vi "StateMachine.vi"() -> ()   [LabVIEW 2021]
uses:
  SynchroCheckCentral.ctl
  SynchroCheckCentral_Info.ctl
  SynchroCheckCentral_Data.ctl
  AFE_froming_Central.ctl
  AFE_froming_Central_Info.ctl
  AFE_froming_Central_Data.ctl
  General Purpose/references.ctl
  Connected_OPF.ctl
  Connected_OPF_Info.ctl
  Connected_OPF_Data.ctl
  Optimal_slack_selection.ctl
  Optimal_slack_selection_Info.ctl
  Optimal_slack_selection_Data.ctl
  State Machine.ctl
panel:
  in  "IN AFE":T1={"Info"={"Resource"="Zenone", "Problem"=FALSE, "Timestamp"=0.0}, "Data"={"Start forming 1"=FALSE, "Forming/Following"=[], "Start forming 2"=FALSE, "measurements"={"Vdc1"=0.0, "P1"=0.0, "Vdc2"=0.0, "P2"=0.0, "Q2"=0.0, "Vdc3"=0.0, "P3"=0.0, "Q3"=0.0, "Vdc4"=0.0, "P4"=0.0, "Q4"=0.0, "Q1"=0.0}, "Status"=[], "references"={"Vdc1"=0.0, "Vdc2"=0.0, "Qac2"=0.0, "Vdc3"=0.0, "Qac3"=0.0, "Vdc4"=0.0, "Qac4"=0.0, "Qac1"=0.0, "V_arg2"=0.0, "V_abs2"=0.0, "V_abs1"=0.0, "V_arg1"=0.0, "freq1"=0.0, "freq2"=0.0}}}
  in  "IN cOPF":T5={"Info"={"Resource"="Zenone", "Problem"=FALSE, "Timestamp"=0.0}, "Data"={"Operation mode"="Grid connected", "solution feasible"=FALSE, "Optimal slack"="AFE 1", "setpoints"=[]}}
  in  "IN iOPF":T5={"Info"={"Resource"="Zenone", "Problem"=FALSE, "Timestamp"=0.0}, "Data"={"Operation mode"="Grid connected", "solution feasible"=FALSE, "Optimal slack"="AFE 1", "setpoints"=[]}}
  in  "IN slack":T8={"Info"={"Resource"="Zenone", "Problem"=FALSE, "Timestamp"=0.0}, "Data"={"Operation mode"="Grid connected", "Optimal slack"="AFE 1", "Time-To-Live"=0.0}}
  in  "IN synchro":T11={"Info"={"Resource"="SyncroCheck", "Problem"=FALSE, "Timestamp"=0.0}, "Data"={"close/open relay"=TRUE, "Operation mode"="Grid connected", "Frequency"=0.0, "Angle"=0.0, "Magnitude"=0.0, "synchronised"=TRUE}}
  out "OUT iOPF":T5={"Info"={"Resource"="Zenone", "Problem"=FALSE, "Timestamp"=0.0}, "Data"={"Operation mode"="Grid connected", "solution feasible"=FALSE, "Optimal slack"="AFE 1", "setpoints"=[]}}
  out "OUT cOPF":T5={"Info"={"Resource"="Zenone", "Problem"=FALSE, "Timestamp"=0.0}, "Data"={"Operation mode"="Grid connected", "solution feasible"=FALSE, "Optimal slack"="AFE 1", "setpoints"=[]}}
  out "OUT AFE":T1={"Info"={"Resource"="Zenone", "Problem"=FALSE, "Timestamp"=0.0}, "Data"={"Start forming 1"=FALSE, "Forming/Following"=[], "Start forming 2"=FALSE, "measurements"={"Vdc1"=0.0, "P1"=0.0, "Vdc2"=0.0, "P2"=0.0, "Q2"=0.0, "Vdc3"=0.0, "P3"=0.0, "Q3"=0.0, "Vdc4"=0.0, "P4"=0.0, "Q4"=0.0, "Q1"=0.0}, "Status"=[], "references"={"Vdc1"=0.0, "Vdc2"=0.0, "Qac2"=0.0, "Vdc3"=0.0, "Qac3"=0.0, "Vdc4"=0.0, "Qac4"=0.0, "Qac1"=0.0, "V_arg2"=0.0, "V_abs2"=0.0, "V_abs1"=0.0, "V_arg1"=0.0, "freq1"=0.0, "freq2"=0.0}}}
  out "OUT Synchro":T11={"Info"={"Resource"="SyncroCheck", "Problem"=FALSE, "Timestamp"=0.0}, "Data"={"close/open relay"=TRUE, "Operation mode"="Grid connected", "Frequency"=0.0, "Angle"=0.0, "Magnitude"=0.0, "synchronised"=TRUE}}
  out "Time-To-Live (minutes)":dbl
  out "setpoints":dbl[](array[numeric])
  in  "nb instances":i16=7
  out "optimal_slack":string(combo)="AFE 1"
  out "iOPF valid":bool
  out "forming?":bool
  out "cOPF valid?":bool
  out "synchronised?":bool
  in  "to grid connection":bool
  in  "to prepare for grid connection":bool
  in  "to island":bool
  in  "Stop":bool
  in  "to prepare for island":bool
  # "Islanding Manoeuvre - State Machine"
  # "synchronised"
  # "opf connected OK"
  # "opf island OK"
  # "forming?"
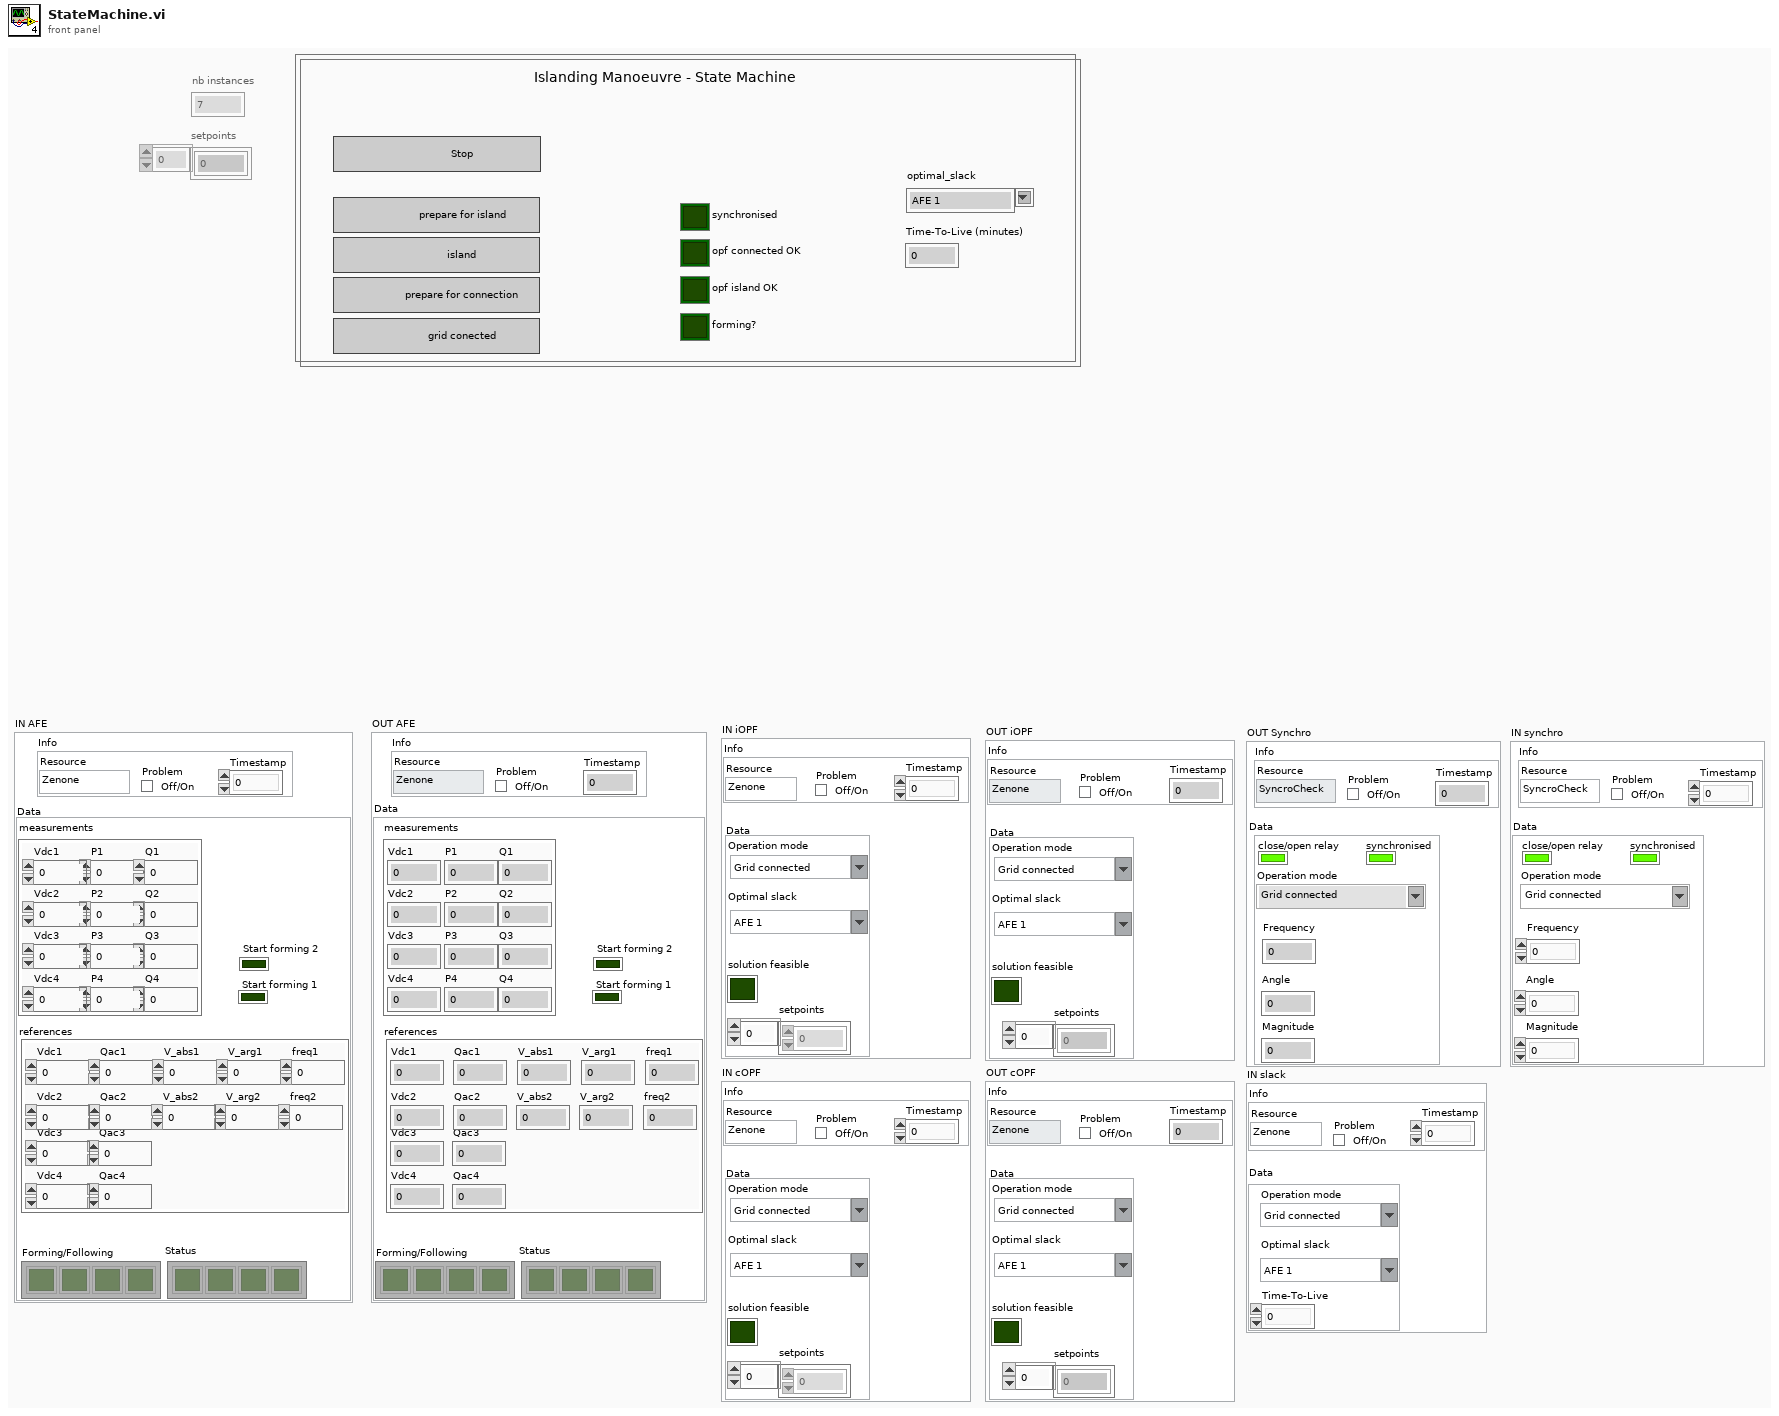
[diagram p1: front panel]
types:
  T1 = typedef "AFE_froming_Central.ctl" = cluster{"Info":T2, "Data":T3}
  T2 = typedef "AFE_froming_Central_Info.ctl" = cluster{"Resource":string, "Problem":bool, "Timestamp":dbl}
  T3 = typedef "AFE_froming_Central_Data.ctl" = cluster{"Start forming 1":bool, "Forming/Following":bool[], "Start forming 2":bool, "measurements":cluster{"Vdc1":dbl, "P1":dbl, "Vdc2":dbl, "P2":dbl, "Q2":dbl, "Vdc3":dbl, "P3":dbl, "Q3":dbl, "Vdc4":dbl, "P4":dbl, "Q4":dbl, "Q1":dbl}, "Status":bool[], "references":T4}
  T4 = typedef "references.ctl" = cluster{"Vdc1":dbl, "Vdc2":dbl, "Qac2":dbl, "Vdc3":dbl, "Qac3":dbl, "Vdc4":dbl, "Qac4":dbl, "Qac1":dbl, "V_arg2":dbl, "V_abs2":dbl, "V_abs1":dbl, "V_arg1":dbl, "freq1":dbl, "freq2":dbl}
  T5 = typedef "Connected_OPF.ctl" = cluster{"Info":T6, "Data":T7}
  T6 = typedef "Connected_OPF_Info.ctl" = cluster{"Resource":string, "Problem":bool, "Timestamp":dbl}
  T7 = typedef "Connected_OPF_Data.ctl" = cluster{"Operation mode":string, "solution feasible":bool, "Optimal slack":string, "setpoints":dbl[]}
  T8 = typedef "Optimal_slack_selection.ctl" = cluster{"Info":T9, "Data":T10}
  T9 = typedef "Optimal_slack_selection_Info.ctl" = cluster{"Resource":string, "Problem":bool, "Timestamp":dbl}
  T10 = typedef "Optimal_slack_selection_Data.ctl" = cluster{"Operation mode":string, "Optimal slack":string, "Time-To-Live":dbl}
  T11 = typedef "SynchroCheckCentral.ctl" = cluster{"Info":T12, "Data":T13}
  T12 = typedef "SynchroCheckCentral_Info.ctl" = cluster{"Resource":string, "Problem":bool, "Timestamp":dbl}
  T13 = typedef "SynchroCheckCentral_Data.ctl" = cluster{"close/open relay":bool, "Operation mode":string, "Frequency":dbl, "Angle":dbl, "Magnitude":dbl, "synchronised":bool}
  T14 = typedef "State Machine.ctl" = enum16{"Grid connected", "Prepare for island", "Island", "Prepare for connection"}
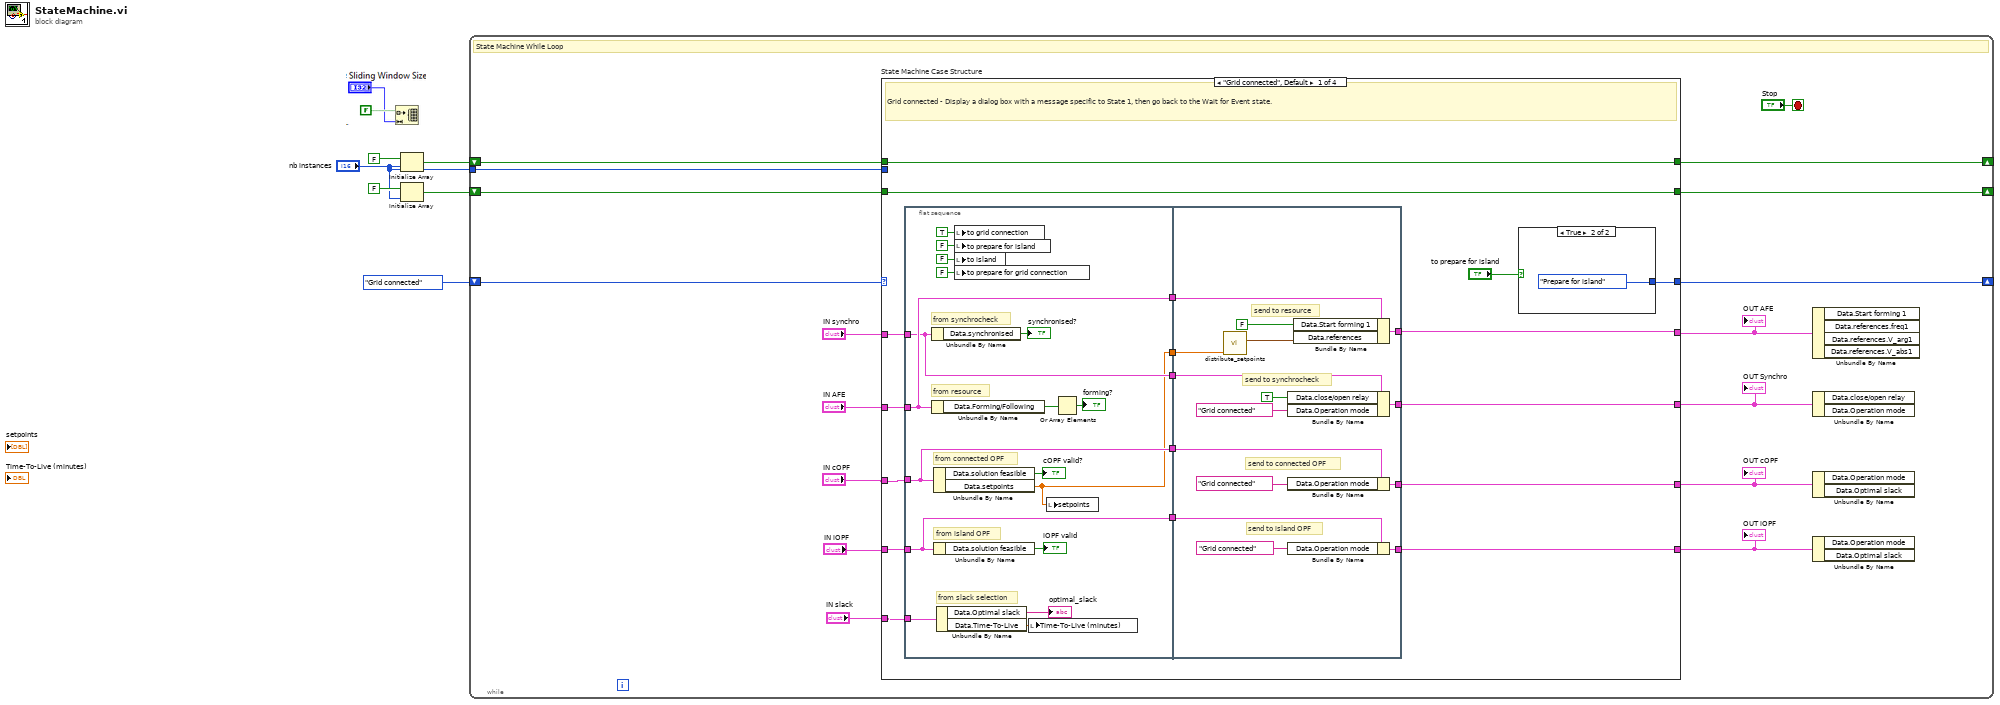
[diagram p0: block diagram]
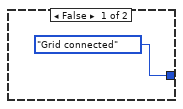
[diagram p2: hidden frame]
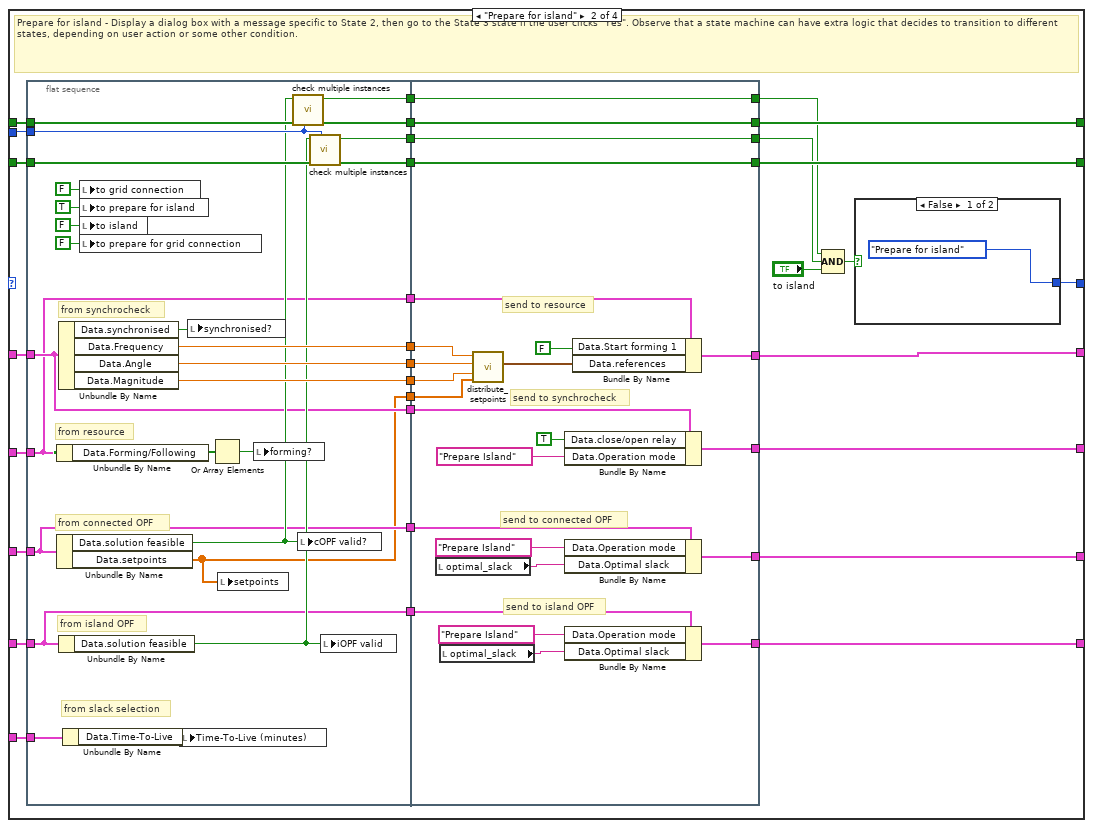
[diagram p3: hidden frame]
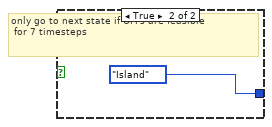
[diagram p4: hidden frame]
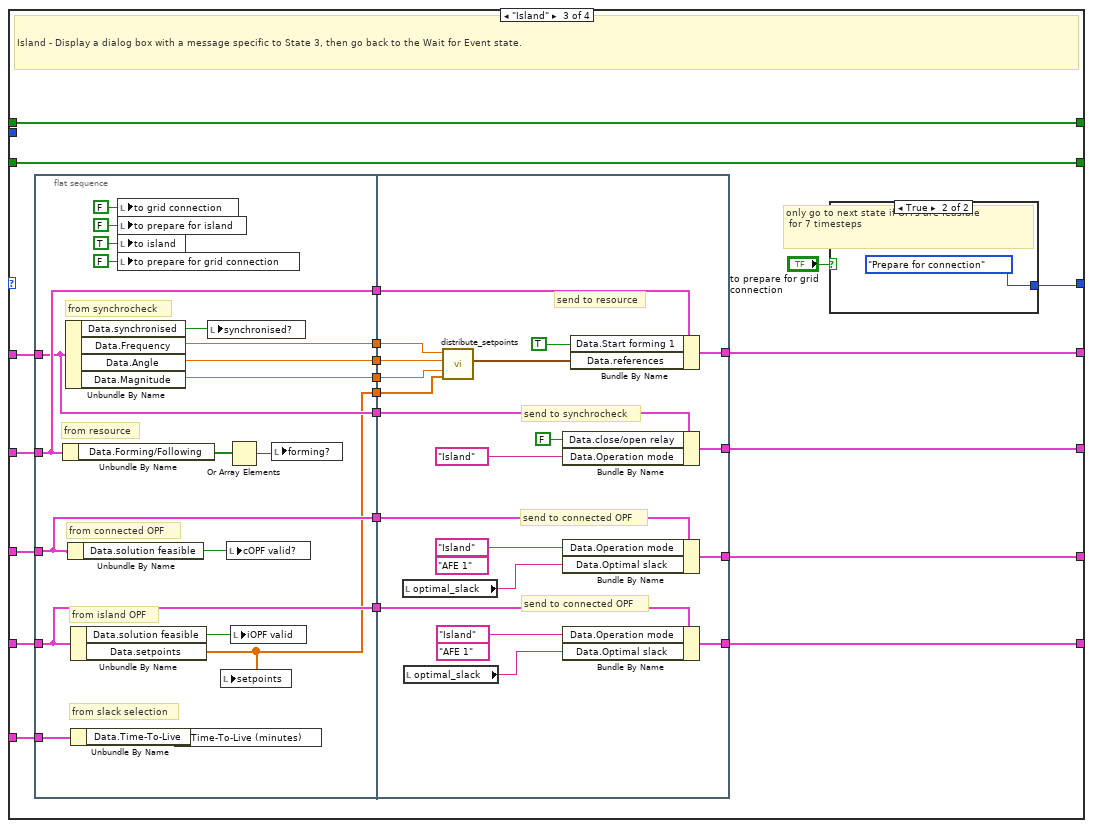
[diagram p5: hidden frame]
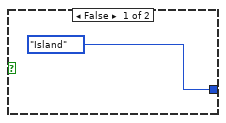
[diagram p6: hidden frame]
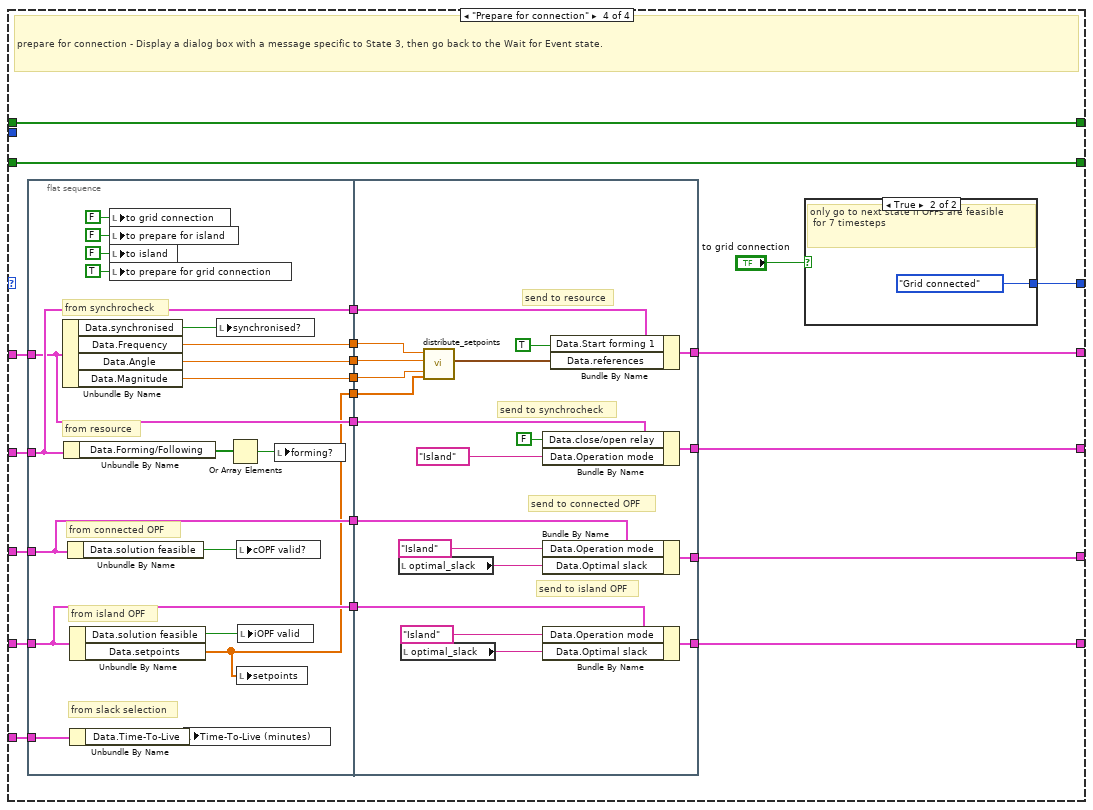
[diagram p7: hidden frame]
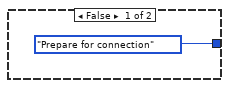
[diagram p8: hidden frame]
diagram:
  n1 = Initialize Array(FALSE, "nb instances") -> (w5:bool[])
  n2 = Initialize Array(FALSE, "nb instances") -> (w3:bool[])
  n3 = while {
    shift-right: [w22] -> _
    shift-left: w5 -> [w23]
    shift-right: [w20] -> _
    shift-left: w3 -> [w21]
    tunnel: "nb instances" -> [w19]
    shift-right: [w12] -> _
    shift-left: State_Machine."Grid connected" ("State") -> [w13]
    stop <- "Stop" stop-if-true
    # "State Machine While Loop"
    n4 = case "State Machine Case Structure" shown="\"Grid connected\", Default" w13 {
      tunnel: "IN synchro" -> [w41 w103 w175 w241]
      tunnel: "IN AFE" -> [w40 w104 w176 w240]
      tunnel: "IN cOPF" -> [w39 w105 w177 w239]
      tunnel: "IN iOPF" -> [w38 w106 w178 w238]
      tunnel: "IN slack" -> [w37 w97 w179 w237]
      tunnel: w23 -> [w36 w102 w174 w236]
      tunnel: [w36 w101 w174 w236] -> w22
      tunnel: w21 -> [w35 w100 w173 w235]
      tunnel: [w35 w99 w173 w235] -> w20
      tunnel: w19 -> [_ w98 _ _]
      tunnel: [w31 w86 w166 w228] -> w18
      tunnel: [w33 w88 w167 w229] -> w17
      tunnel: [w32 w87 w168 w230] -> w16
      tunnel: [w34 w89 w169 w231] -> w15
      tunnel: [w29 w81 w164 w226] -> w12
      frame "Grid connected", Default {
        # "Grid connected - Display a dialog box with a message specific to State 1, then go back to the Wait for Event state."
        n5 = flat-sequence {
          tunnel: w41 -> [w48]
          tunnel: w40 -> [w49]
          tunnel: w39 -> [w47]
          tunnel: w38 -> [w46]
          tunnel: w37 -> [w50]
          tunnel: [w49] -> w28
          tunnel: [w48] -> w27
          tunnel: [w47] -> w26
          tunnel: [w46] -> w25
          tunnel: [w44] -> w24
          tunnel: [w70] -> w34
          tunnel: [w69] -> w33
          tunnel: [w68] -> w32
          tunnel: [w67] -> w31
          tunnel: w28 -> [w66]
          tunnel: w27 -> [w65]
          tunnel: w26 -> [w64]
          tunnel: w25 -> [w63]
          tunnel: w24 -> [w61]
          frame #0 {
            # "from slack selection"
            # "from island OPF"
            # "from connected OPF"
            # "from resource"
            # "from synchrocheck"
            n6 = Unbundle By Name(w48) -> ("Data.synchronised"=→"synchronised?":bool)
            n7 = Unbundle By Name(w49) -> ("Data.Forming/Following"=w57:bool[])
            n8 = Unbundle By Name(w47) -> ("Data.solution feasible"=→"cOPF valid?":bool, "Data.setpoints"=w44:dbl[])
            n9 = Unbundle By Name(w46) -> ("Data.solution feasible"=→"iOPF valid":bool)
            n10 = Unbundle By Name(w50) -> ("Data.Optimal slack"=→"optimal_slack":string, "Data.Time-To-Live"=w45:dbl)
            n11 = local write "to grid connection"(TRUE ("to grid connection")) -> ()
            n12 = local write "to prepare for island"(FALSE ("to prepare for island")) -> ()
            n13 = local write "to island"(FALSE ("to island")) -> ()
            n14 = local write "to prepare for grid connection"(FALSE ("to prepare for grid connection")) -> ()
            n15 = local write "Time-To-Live (minutes)"(w45) -> ()
            n16 = local write "setpoints"(w44) -> ()
            n17 = Or Array Elements(Boolean array=w57) -> (logical OR=→"forming?":bool)
          }
          frame #1 {
            # "send to island OPF"
            # "send to resource"
            # "send to connected OPF"
            # "send to synchrocheck"
            n18 = call "distribute_setpoints.vi"("setpoints"=w61) -> ("references"=w62:T4)  [unwired: 10 in]
            n19 = Bundle By Name(cluster=w65, "Data.close/open relay"=TRUE, "Data.Operation mode"="Grid connected" ("Operation mode")) -> (w67:T11)
            n20 = Bundle By Name(cluster=w64, "Data.Operation mode"="Grid connected" ("Operation mode")) -> (w68:T5)
            n21 = Bundle By Name(cluster=w63, "Data.Operation mode"="Grid connected" ("Operation mode")) -> (w70:T5)
            n22 = Bundle By Name(cluster=w66, "Data.Start forming 1"=FALSE, "Data.references"=w62) -> (w69:T1)
          }
        }
        n23 = case shown="True" "to prepare for island" {
          tunnel: [State_Machine."Grid connected" ("State") State_Machine."Prepare for island" ("State")] -> w29
          frame False {
          }
          frame True {
          }
        }
      }
      frame "Prepare for island" {
        # "Prepare for island - Display a dialog box with a message specific to State 2, then go to the State 3 state if the user clicks \"Yes\". Observe that a state machine can have extra logic that decides to transition to different states, depending on user action or some other condition."
        n24 = flat-sequence {
          tunnel: w106 -> [w113]
          tunnel: w105 -> [w112]
          tunnel: w104 -> [w110]
          tunnel: w103 -> [w111]
          tunnel: w102 -> [w130]
          tunnel: w100 -> [w128]
          tunnel: w98 -> [w124]
          tunnel: w97 -> [w123]
          tunnel: [w133] -> w96
          tunnel: [w132] -> w95
          tunnel: [w131] -> w94
          tunnel: [w129] -> w93
          tunnel: [w127] -> w92
          tunnel: [w126] -> w91
          tunnel: [w125] -> w90
          tunnel: [w113] -> w80
          tunnel: [w112] -> w79
          tunnel: [w111] -> w78
          tunnel: [w110] -> w77
          tunnel: [w109] -> w76
          tunnel: w96 -> [w138]
          tunnel: w95 -> [w137]
          tunnel: w94 -> [w136]
          tunnel: w93 -> [w158]
          tunnel: w92 -> [w157]
          tunnel: w91 -> [w145]
          tunnel: w90 -> [w144]
          tunnel: [w158] -> w101
          tunnel: [w157] -> w99
          tunnel: [w149] -> w89
          tunnel: [w148] -> w88
          tunnel: [w147] -> w87
          tunnel: [w146] -> w86
          tunnel: [w144] -> w83
          tunnel: [w145] -> w82
          tunnel: w80 -> [w143]
          tunnel: w79 -> [w142]
          tunnel: w78 -> [w141]
          tunnel: w77 -> [w140]
          tunnel: w76 -> [w135]
          frame #0 {
            # "from slack selection"
            # "from island OPF"
            # "from connected OPF"
            # "from resource"
            # "from synchrocheck"
            n25 = Unbundle By Name(w110) -> ("Data.Forming/Following"=w134:bool[])
            n26 = Unbundle By Name(w112) -> ("Data.solution feasible"=w115:bool, "Data.setpoints"=w109:dbl[])
            n27 = Unbundle By Name(w111) -> ("Data.synchronised"=w117:bool, "Data.Frequency"=w133:dbl, "Data.Angle"=w132:dbl, "Data.Magnitude"=w131:dbl)
            n28 = Unbundle By Name(w113) -> ("Data.solution feasible"=w114:bool)
            n29 = Unbundle By Name(w123) -> ("Data.Time-To-Live"=w122:dbl)
            n30 = local write "to grid connection"(FALSE ("to grid connection")) -> ()
            n31 = local write "to prepare for island"(TRUE ("to prepare for island")) -> ()
            n32 = local write "to island"(FALSE ("to island")) -> ()
            n33 = local write "to prepare for grid connection"(FALSE ("to prepare for grid connection")) -> ()
            n34 = local write "Time-To-Live (minutes)"(w122) -> ()
            n35 = local write "synchronised?"(w117) -> ()
            n36 = Or Array Elements(Boolean array=w134) -> (logical OR=w116:bool)
            n37 = local write "setpoints"(w109) -> ()
            n38 = local write "forming?"(w116) -> ()
            n39 = call "check multiple instances.vi"("nb instances"=w124, "array elements in"=w130, "new element"=w115) -> ("array elements out"=w129:bool[], "out"=w125:bool)  [unwired: 7 in]
            n40 = local write "cOPF valid?"(w115) -> ()
            n41 = call "check multiple instances.vi"("nb instances"=w124, "array elements in"=w128, "new element"=w114) -> ("array elements out"=w127:bool[], "out"=w126:bool)  [unwired: 7 in]
            n42 = local write "iOPF valid"(w114) -> ()
          }
          frame #1 {
            # "send to island OPF"
            # "send to resource"
            # "send to connected OPF"
            # "send to synchrocheck"
            n43 = local read "optimal_slack"() -> (w155:string)
            n44 = local read "optimal_slack"() -> (w156:string)
            n45 = call "distribute_setpoints.vi"("setpoints"=w135, "Magnitude"=w136, "Angle"=w137, "Frequency"=w138) -> ("references"=w139:T4)  [unwired: 7 in]
            n46 = Bundle By Name(cluster=w141, "Data.close/open relay"=TRUE, "Data.Operation mode"="Prepare Island" ("Operation mode")) -> (w146:T11)
            n47 = Bundle By Name(cluster=w142, "Data.Operation mode"="Prepare Island" ("Operation mode"), "Data.Optimal slack"=w155) -> (w147:T5)
            n48 = Bundle By Name(cluster=w143, "Data.Operation mode"="Prepare Island" ("Operation mode"), "Data.Optimal slack"=w156) -> (w149:T5)
            n49 = Bundle By Name(cluster=w140, "Data.Start forming 1"=FALSE, "Data.references"=w139) -> (w148:T1)
          }
        }
        n50 = Compound Arithmetic op=AND(w83, w82, "to island") -> (w85:bool)
        n51 = case shown="False" w85 {
          tunnel: [State_Machine."Prepare for island" ("State") State_Machine."Island" ("State")] -> w81
          frame False {
          }
          frame True {
            # "only go to next state if OPFs are feasible\n for 7 timesteps"
          }
        }
      }
      frame "Island" {
        # "Island - Display a dialog box with a message specific to State 3, then go back to the Wait for Event state."
        n52 = flat-sequence {
          tunnel: w179 -> [w196]
          tunnel: w178 -> [w186]
          tunnel: w177 -> [w185]
          tunnel: w176 -> [w184]
          tunnel: w175 -> [w183]
          tunnel: [w199] -> w172
          tunnel: [w198] -> w171
          tunnel: [w197] -> w170
          tunnel: [w186] -> w163
          tunnel: [w185] -> w162
          tunnel: [w184] -> w161
          tunnel: [w183] -> w160
          tunnel: [w182] -> w159
          tunnel: w172 -> [w203]
          tunnel: w171 -> [w204]
          tunnel: w170 -> [w205]
          tunnel: [w213] -> w169
          tunnel: [w212] -> w168
          tunnel: [w211] -> w167
          tunnel: [w210] -> w166
          tunnel: w163 -> [w209]
          tunnel: w162 -> [w208]
          tunnel: w161 -> [w207]
          tunnel: w160 -> [w206]
          tunnel: w159 -> [w201]
          frame #0 {
            # "from slack selection"
            # "from island OPF"
            # "from connected OPF"
            # "from resource"
            # "from synchrocheck"
            n53 = Unbundle By Name(w184) -> ("Data.Forming/Following"=w200:bool[])
            n54 = Unbundle By Name(w183) -> ("Data.synchronised"=w190:bool, "Data.Frequency"=w197:dbl, "Data.Angle"=w198:dbl, "Data.Magnitude"=w199:dbl)
            n55 = Unbundle By Name(w185) -> ("Data.solution feasible"=w188:bool)
            n56 = Unbundle By Name(w186) -> ("Data.solution feasible"=w187:bool, "Data.setpoints"=w182:dbl[])
            n57 = Unbundle By Name(w196) -> ("Data.Time-To-Live"=w195:dbl)
            n58 = local write "to grid connection"(FALSE ("to grid connection")) -> ()
            n59 = local write "to prepare for island"(FALSE ("to prepare for island")) -> ()
            n60 = local write "to island"(TRUE ("to island")) -> ()
            n61 = local write "to prepare for grid connection"(FALSE ("to prepare for grid connection")) -> ()
            n62 = local write "Time-To-Live (minutes)"(w195) -> ()
            n63 = local write "synchronised?"(w190) -> ()
            n64 = local write "setpoints"(w182) -> ()
            n65 = local write "cOPF valid?"(w188) -> ()
            n66 = Or Array Elements(Boolean array=w200) -> (logical OR=w189:bool)
            n67 = local write "iOPF valid"(w187) -> ()
            n68 = local write "forming?"(w189) -> ()
          }
          frame #1 {
            (unwired) "AFE 1" ("Optimal slack")
            (unwired) "AFE 1" ("Optimal slack")
            # "send to connected OPF"
            # "send to connected OPF"
            # "send to resource"
            # "send to synchrocheck"
            n69 = local read "optimal_slack"() -> (w219:string)
            n70 = local read "optimal_slack"() -> (w220:string)
            n71 = call "distribute_setpoints.vi"("setpoints"=w201, "Magnitude"=w203, "Angle"=w204, "Frequency"=w205) -> ("references"=w202:T4)  [unwired: 7 in]
            n72 = Bundle By Name(cluster=w206, "Data.close/open relay"=FALSE, "Data.Operation mode"="Island" ("Operation mode")) -> (w210:T11)
            n73 = Bundle By Name(cluster=w208, "Data.Operation mode"="Island" ("Operation mode"), "Data.Optimal slack"=w219) -> (w212:T5)
            n74 = Bundle By Name(cluster=w209, "Data.Operation mode"="Island" ("Operation mode"), "Data.Optimal slack"=w220) -> (w213:T5)
            n75 = Bundle By Name(cluster=w207, "Data.Start forming 1"=TRUE, "Data.references"=w202) -> (w211:T1)
          }
        }
        n76 = case shown="True" "to prepare for grid connection" {
          tunnel: [State_Machine."Island" ("State") State_Machine."Prepare for connection" ("State")] -> w164
          frame False {
          }
          frame True {
            # "only go to next state if OPFs are feasible\n for 7 timesteps"
          }
        }
      }
      frame "Prepare for connection" {
        # "prepare for connection - Display a dialog box with a message specific to State 3, then go back to the Wait for Event state."
        n77 = flat-sequence {
          tunnel: w241 -> [w245]
          tunnel: w240 -> [w246]
          tunnel: w239 -> [w247]
          tunnel: w238 -> [w248]
          tunnel: w237 -> [w258]
          tunnel: [w261] -> w234
          tunnel: [w260] -> w233
          tunnel: [w259] -> w232
          tunnel: [w248] -> w225
          tunnel: [w247] -> w224
          tunnel: [w246] -> w223
          tunnel: [w245] -> w222
          tunnel: [w244] -> w221
          tunnel: w234 -> [w264]
          tunnel: w233 -> [w265]
          tunnel: w232 -> [w266]
          tunnel: [w275] -> w231
          tunnel: [w274] -> w230
          tunnel: [w273] -> w229
          tunnel: [w272] -> w228
          tunnel: w225 -> [w271]
          tunnel: w224 -> [w270]
          tunnel: w223 -> [w269]
          tunnel: w222 -> [w268]
          tunnel: w221 -> [w263]
          frame #0 {
            # "from slack selection"
            # "from island OPF"
            # "from connected OPF"
            # "from resource"
            # "from synchrocheck"
            n78 = Unbundle By Name(w245) -> ("Data.synchronised"=w252:bool, "Data.Frequency"=w259:dbl, "Data.Angle"=w260:dbl, "Data.Magnitude"=w261:dbl)
            n79 = Unbundle By Name(w246) -> ("Data.Forming/Following"=w262:bool[])
            n80 = Unbundle By Name(w247) -> ("Data.solution feasible"=w250:bool)
            n81 = Unbundle By Name(w248) -> ("Data.solution feasible"=w249:bool, "Data.setpoints"=w244:dbl[])
            n82 = Unbundle By Name(w258) -> ("Data.Time-To-Live"=w257:dbl)
            n83 = local write "to grid connection"(FALSE ("to grid connection")) -> ()
            n84 = local write "to prepare for island"(FALSE ("to prepare for island")) -> ()
            n85 = local write "to island"(FALSE ("to island")) -> ()
            n86 = local write "to prepare for grid connection"(TRUE ("to prepare for grid connection")) -> ()
            n87 = local write "Time-To-Live (minutes)"(w257) -> ()
            n88 = local write "synchronised?"(w252) -> ()
            n89 = Or Array Elements(Boolean array=w262) -> (logical OR=w251:bool)
            n90 = local write "cOPF valid?"(w250) -> ()
            n91 = local write "setpoints"(w244) -> ()
            n92 = local write "iOPF valid"(w249) -> ()
            n93 = local write "forming?"(w251) -> ()
          }
          frame #1 {
            # "send to island OPF"
            # "send to connected OPF"
            # "send to resource"
            # "send to synchrocheck"
            n94 = local read "optimal_slack"() -> (w281:string)
            n95 = local read "optimal_slack"() -> (w282:string)
            n96 = call "distribute_setpoints.vi"("setpoints"=w263, "Magnitude"=w264, "Angle"=w265, "Frequency"=w266) -> ("references"=w267:T4)  [unwired: 7 in]
            n97 = Bundle By Name(cluster=w268, "Data.close/open relay"=FALSE, "Data.Operation mode"="Island" ("Operation mode")) -> (w272:T11)
            n98 = Bundle By Name(cluster=w270, "Data.Operation mode"="Island" ("Operation mode"), "Data.Optimal slack"=w281) -> (w274:T5)
            n99 = Bundle By Name(cluster=w271, "Data.Operation mode"="Island" ("Operation mode"), "Data.Optimal slack"=w282) -> (w275:T5)
            n100 = Bundle By Name(cluster=w269, "Data.Start forming 1"=TRUE, "Data.references"=w267) -> (w273:T1)
          }
        }
        n101 = case shown="True" "to grid connection" {
          tunnel: [State_Machine."Prepare for connection" ("State") State_Machine."Grid connected" ("State")] -> w226
          frame False {
          }
          frame True {
            # "only go to next state if OPFs are feasible\n for 7 timesteps"
          }
        }
      }
    }
    "OUT Synchro" <- w18
    "OUT AFE" <- w17
    "OUT cOPF" <- w16
    "OUT iOPF" <- w15
    n102 = Unbundle By Name(w17) -> ()  [unwired: 4 out]
    n103 = Unbundle By Name(w18) -> ()  [unwired: 2 out]
    n104 = Unbundle By Name(w16) -> ()  [unwired: 2 out]
    n105 = Unbundle By Name(w15) -> ()  [unwired: 2 out]
  }
